vi "Calculate Plot Range.vi"(8 "error in (no error)":errorcluster, 9 "Coordinates System":enum16{"Cartesian", "Cylindrical", "Spherical"}(ring), 10 "3D Pie Datatype.lvclass in":refnum<class "3D Pie Datatype.lvclass">, 11 "Plot Representation In":T1) -> (0 "error out":errorcluster, 2 "3D Pie Datatype.lvclass out":refnum<class "3D Pie Datatype.lvclass">, 3 "Plot Representation Out":T1)   [LabVIEW 2017, in "3D Pie Datatype.lvclass"]
uses:
  <vilib>/Math Plots/3D Math Plots/3D Pie/3D Pie Datatype/3D Pie Datatype.lvclass
  <vilib>/Math Plots/3D Math Plots/3D Plot/3D Plot/Typedef/Plot Representation.ctl
  <vilib>/Math Plots/3D Math Plots/3D Plot/3D Plot/Typedef/Range Clusters.ctl
  <vilib>/Math Plots/3D Math Plots/3D Plot/3D Plot/Typedef/Mesh Data.ctl
  <vilib>/Math Plots/3D Math Plots/3D Plot/3D Plot/3D Plot.lvclass
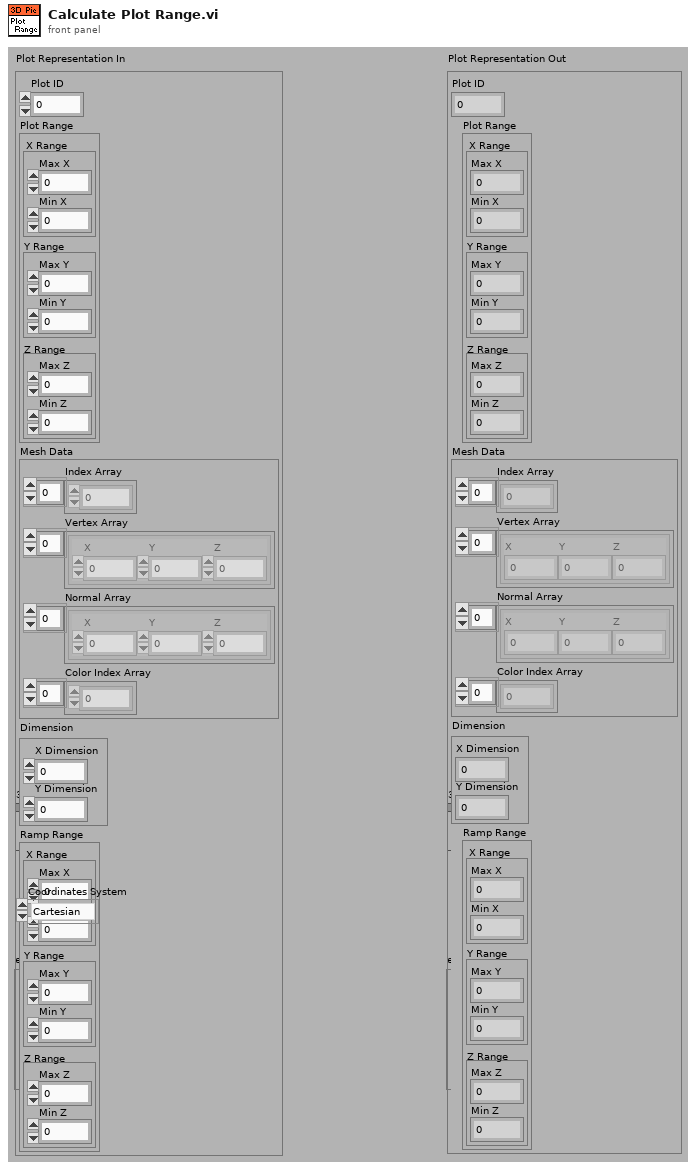
[diagram p1: front panel]
types:
  T1 = typedef "3D Plot.lvclass/Plot Representation.ctl" = cluster{"Plot ID":i32, "Plot Range":T2, "Mesh Data":T3, "Dimension":cluster{"X Dimension":i32, "Y Dimension":i32}, "Ramp Range":T2}
  T2 = typedef "3D Plot.lvclass/Range Clusters.ctl" = cluster{"X Range":cluster{"Max X":sgl, "Min X":sgl}, "Y Range":cluster{"Max Y":sgl, "Min Y":sgl}, "Z Range":cluster{"Max Z":sgl, "Min Z":sgl}}
  T3 = typedef "3D Plot.lvclass/Mesh Data.ctl" = cluster{"Index Array":u32[], "Vertex Array":cluster{"X":sgl, "Y":sgl, "Z":sgl}[], "Normal Array":cluster{"X":sgl, "Y":sgl, "Z":sgl}[], "Color Index Array":i32[]}
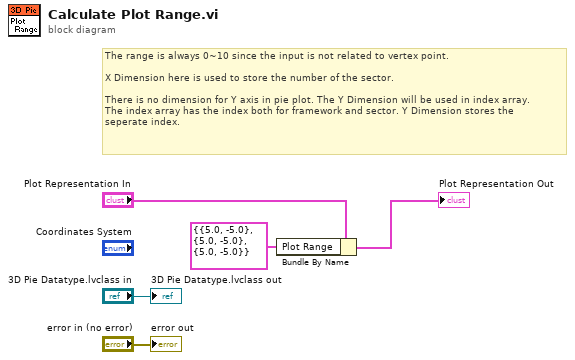
[diagram p0: block diagram]
diagram:
  # "The range is always 0~10 since the input is not related to vertex point.\n\nX Dimension here is used to store the number of the sector.\n\nThere is no dimension for Y axis in pie plot. The Y Dimension will be used in index array.\nThe index array has the index both for framework and sector. Y Dimension stores the \nseperate index."
  n1 = Bundle By Name(cluster="Plot Representation In", "Plot Range"=T2 {"X Range"={"Max X"=5.0, "Min X"=-5.0}, "Y Range"={"Max Y"=5.0, "Min Y"=-5.0}, "Z Range"={"Max Z"=5.0, "Min Z"=-5.0}} ("This Range Min/Max Out")) -> (→"Plot Representation Out":T1)
  "error out" <- "error in (no error)"
  "3D Pie Datatype.lvclass out" <- "3D Pie Datatype.lvclass in"
